vi "Read String.vi"(8 "error in (no error)":errorcluster, 11 "ContextData in":refnum<class "ContextData.lvclass">) -> (0 "error out":errorcluster, 2 "String <Replace Me>":string, 3 "ContextData out":refnum<class "ContextData.lvclass">)   [LabVIEW 2019]
uses:
  ContextData.lvclass
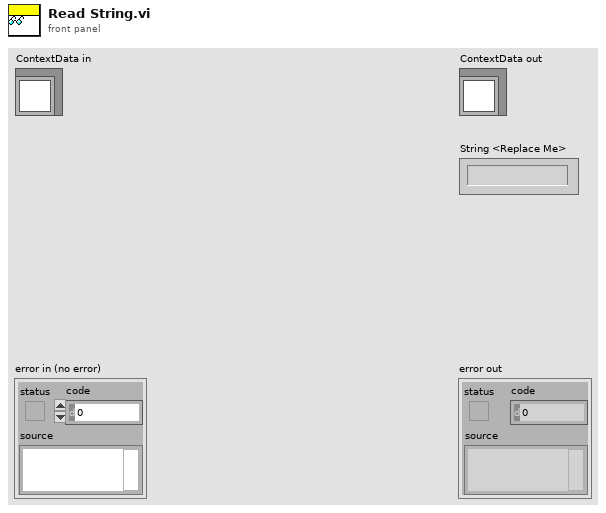
[diagram p1: front panel]
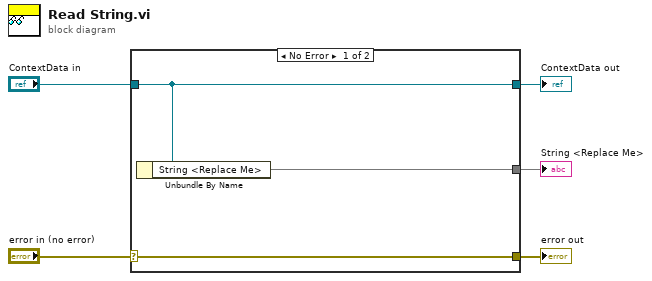
[diagram p0: block diagram]
diagram:
  n1 = case shown="No Error" "error in (no error)" {
    selector: "error in (no error)" -> [w8 w9]
    tunnel: [w8 w9] -> w4
    tunnel: [w7 w10] -> w2
    tunnel: "ContextData in" -> [w7 w10]
    tunnel: [w6 _] -> w1
    frame No Error {
      n2 = Unbundle By Name(w7) -> ("String <Replace Me>"=w6)
    }
    frame Error {
    }
  }
  "error out" <- w4
  "ContextData out" <- w2
  "String <Replace Me>" <- w1
